vi "populateEventSettingVersions.vi"(8 "error in (no error)":errorcluster, 11 "Model in":refnum<class "Model.lvclass">) -> (0 "error out":errorcluster, 3 "Model out":refnum<class "Model.lvclass">)   [LabVIEW 2016, in "Model.lvclass"]
uses:
  Model.lvclass
  Model.lvclass/Model.ctl
  Publisher/Publisher.lvclass/Publisher.ctl
  Publisher/Publisher.lvclass
  Boot/Boot.lvclass
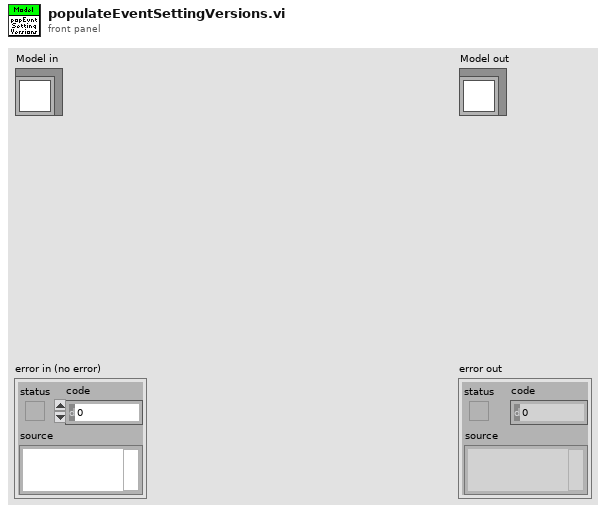
[diagram p1: front panel]
types:
  T1 = typedef "M1M3SupportSettings.lvlib/RecommendedSettings.ctl" = cluster{"RecommendedSettings":string[]}
  T2 = typedef "M1M3SupportTopics.lvlib/Timestamp.ctl" = dbl
  T3 = typedef "M1M3SupportTopics.lvlib/EventSettingVersions.ctl" = cluster{"Timestamp":T2, "RecommendedSettingsVersion":string}
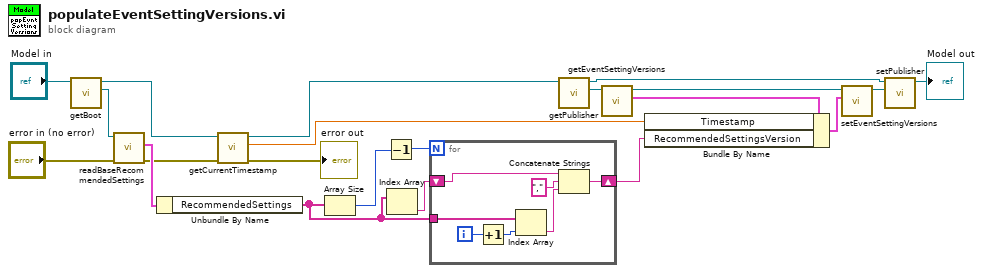
[diagram p0: block diagram]
diagram:
  n1 = call "getBoot.vi"("Model in"="Model in") -> ("Boot"=w11:refnum<class "Boot.lvclass">, "Model out"=w10:refnum<class "Model.lvclass">)  [unwired: 9 in]
  n2 = call "readBaseRecommendedSettings.vi"("error in (no error)"="error in (no error)", "Boot in"=w11) -> ("error out"=w2:errorcluster, "RecommendedSettings"=w9:T1)  [unwired: 7 in, 1 out]
  n3 = Unbundle By Name(w9) -> ("RecommendedSettings"=w7:string[])
  n4 = call "getCurrentTimestamp.vi"("error in (no error)"=w2, "Model in"=w10) -> ("error out"=→"error out":errorcluster, "Timestamp"=w15:T2, "Model out"=w21:refnum<class "Model.lvclass">)  [unwired: 7 in]
  n5 = Array Size(array=w7) -> (size(s)=w8:i32)
  n6 = Decrement(x=w8) -> (x-1=w6:i32)
  n7 = Index Array(array=w7) -> (element=w5:string)  [unwired: 1 in]
  n8 = for {
    N: w6 -> [_]
    tunnel: w7 -> [w26]
    shift-right: [w25] -> w4
    shift-left: w5 -> [w24]
    i -> [w28]
    n9 = Increment(x=w28) -> (x+1=w27:i32)
    n10 = Index Array(array=w26, index=w27) -> (element=w22:string)
    n11 = Concatenate Strings(w24, "," ("string"), w22) -> (w25:string)
  }
  n12 = call "getPublisher.vi"("Model in"=w21) -> ("Publisher"=w18:refnum<class "Publisher.lvclass">, "Model out"=w20:refnum<class "Model.lvclass">)  [unwired: 9 in]
  n13 = call "getEventSettingVersions.vi"("Publisher in"=w18) -> ("EventSettingVersions"=w17:T3, "Publisher out"=w13:refnum<class "Publisher.lvclass">)  [unwired: 9 in]
  n14 = Bundle By Name(cluster=w17, "Timestamp"=w15, "RecommendedSettingsVersion"=w4) -> (w16:T3)
  n15 = call "setEventSettingVersions.vi"("EventSettingVersions"=w16, "Publisher in"=w13) -> ("Publisher out"=w14:refnum<class "Publisher.lvclass">)  [unwired: 9 in]
  n16 = call "setPublisher.vi"("Publisher"=w14, "Model in"=w20) -> ("Model out"=→"Model out":refnum<class "Model.lvclass">)  [unwired: 9 in]
